vi "SiosIfmAngleAvailable.vi"(1 "Channel2":i32(knob) scale=1.0..4.0, 2 "Channel1":i32(knob) scale=1.0..4.0, 3 "Device Number":i32) -> (0 "Success":i32)   [LabVIEW 2009]
uses:
  siosifm.dll
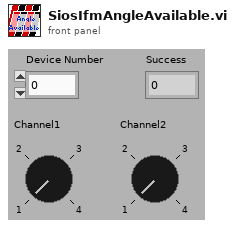
[diagram p1: front panel]
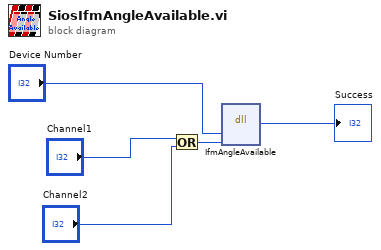
[diagram p0: block diagram]
diagram:
  n1 = Or(x="Channel1", y="Channel2") -> (x .or. y?=w3:i32)
  n2 = dll-call lib="C:/WORK/Artem/RE-10/SIOS_IfmDLL/siosifm.dll" fn="IfmAngleAvailable"("devNumber"="Device Number", "channelmask"=w3) -> ("Success"=→"Success":i32)  [unwired: 5 in, 2 out]
